vi "GetNoteFromLineHTML.vi"(10 "Regular Expression (Separator)":string, 11 "HTML Line":string) -> (3 "String out":string)   [LabVIEW 2018, in "DS_Lib.lvlib" / "SRNotesParser.lvlib"]
uses:
  SRNotesParser.lvlib
  <userlib>/_OpenG.lib/string/string.llb/Trim Whitespace (String)__ogtk.vi
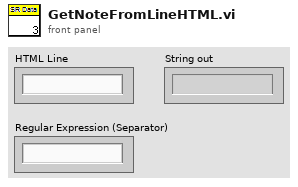
[diagram p1: front panel]
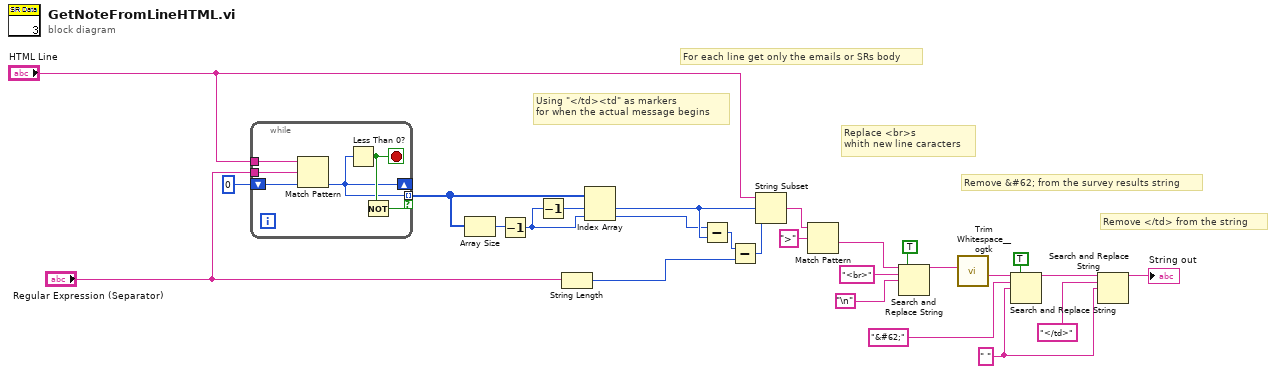
[diagram p0: block diagram]
diagram:
  w2 = " " ("replace string (\"\")")
  # "Remove </td> from the string"
  # "Remove &#62; from the survey results string"
  # "Replace <br>s \nwhith new line caracters"
  # "Using \"</td><td\" as markers \nfor when the actual message begins"
  # "For each line get only the emails or SRs body"
  n1 = while {
    tunnel: [w29] -> w10 mode=indexing if=w31
    tunnel: "HTML Line" -> [w30]
    shift-right: [w29] -> _
    shift-left: 0 ("offset past match") -> [w28]
    tunnel: "Regular Expression (Separator)" -> [w27]
    stop <- w32 stop-if-true
    n2 = Match Pattern(string=w30, regular expression=w27, offset (0)=w28) -> (offset past match=w29:i32)  [unwired: 3 out]
    n3 = Less Than 0?(x=w29) -> (x < 0?=w32:bool)
    n4 = Not(x=w32) -> (.not. x?=w31:bool)
  }
  n5 = Array Size(array=w10) -> (size(s)=w11:i32)
  n6 = Decrement(x=w11) -> (x-1=w19:i32)
  n7 = Decrement(x=w19) -> (x-1=w18:i32)
  n8 = String Length(string="Regular Expression (Separator)") -> (length=w25:i32)
  n9 = Index Array(array=w10, index #1=w18, index #2=w19) -> (element #1=w21:i32, element #2=w20:i32)
  n10 = Subtract(x=w20, y=w21) -> (x-y=w22:i32)
  n11 = Subtract(x=w22, y=w25) -> (x-y=w23:i32)
  n12 = String Subset(string="HTML Line", offset (0)=w21, length (rest)=w23) -> (substring=w9:string)
  n13 = Match Pattern(string=w9, regular expression=">") -> (after substring=w8:string)  [unwired: 1 in, 3 out]
  n14 = Search and Replace String(replace all?=TRUE ("replace all? (F)"), input string=w8, search string="<br>", replace string="\n") -> (result string=w24:string)  [unwired: 4 in, 3 out]
  n15 = call-poly <userlib>:"Trim Whitespace__ogtk.vi"("String in"=w24) -> ("String out"=w7:string)  [unwired: 6 in]
  n16 = Search and Replace String(replace all?=TRUE ("replace all? (F)"), input string=w7, search string="&#62;", replace string=w2) -> (result string=w4:string)  [unwired: 4 in, 3 out]
  n17 = Search and Replace String(input string=w4, search string="</td>", replace string=w2) -> (result string=→"String out":string)  [unwired: 5 in, 3 out]
